vi "WritePFIReport_TempTest.vi"(8 "error in (no error)":errorcluster, 11 "Temp PFI":string[][][](array[string])=[[["11", "12"], ["11", "12"], ["11", "12"], ["11", "12"], ["11", "12"], ["11", "12"], ["11", ""], ["11", ""], ["11", ""], ["11", ""], ["11", ""], ["11", ""], ["", ""], ["", ""]], [["21", "22"], ["21", "22"], ["21", "22"], ["21", "22"], ["21", "22"], ["21", "22"], ["21", "22"], ["21", "22"], ["21", "22"], ["21", "22"], ["21", "22"], ["21", "22"], ["21", "22"], ["21", "22"]]]) -> (0 "error in (no error) 2":errorcluster)   [LabVIEW 2014]
uses:
  Excel(ActiveX)/enumOpenOrCreate.ctl
  Excel(ActiveX)/Excel(ActiveX).lvlib
panel:
  out "deleted portion":string[][](array[string])
  out "array w/ subset deleted":string[][](array[string])
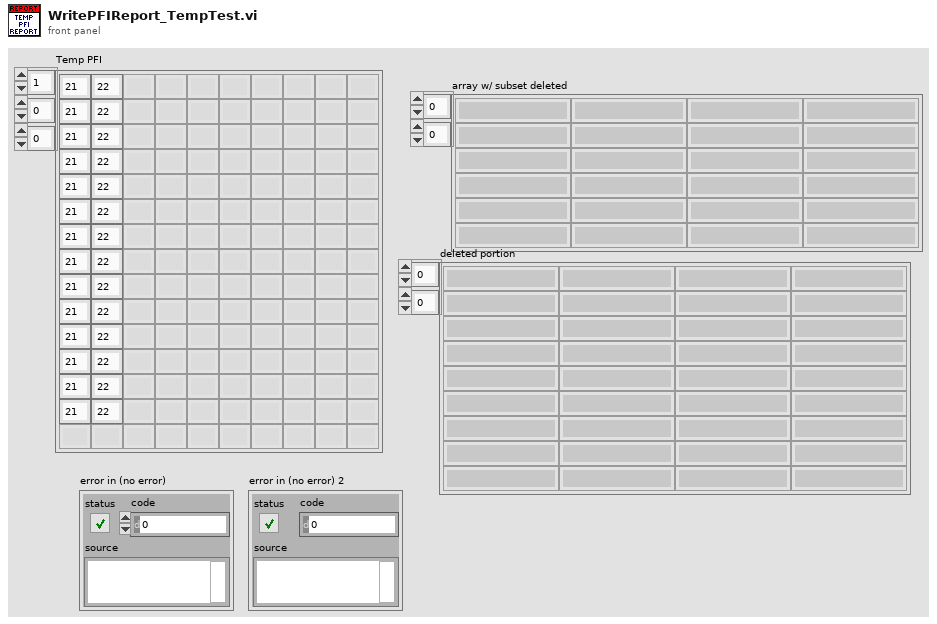
[diagram p1: front panel]
types:
  T1 = typedef "Excel(ActiveX).lvlib/enumOpenOrCreate.ctl" = enum16{"open", "open or create", "create from template"}
  T2 = typedef "Excel(ActiveX).lvlib/ExcelActiveX.ctl" = cluster{"Excel._Application":refnum<k7>, "Application open at start":bool, "Excel._Worksheet":refnum<k7>, "Workbook open at start":bool, "Excel._Workbook":refnum<k7>, "Workbook Path":path, "Worksheet Name":string, "Row":u32, "Col":u32, "Cell":string, "Workbook Name":string}
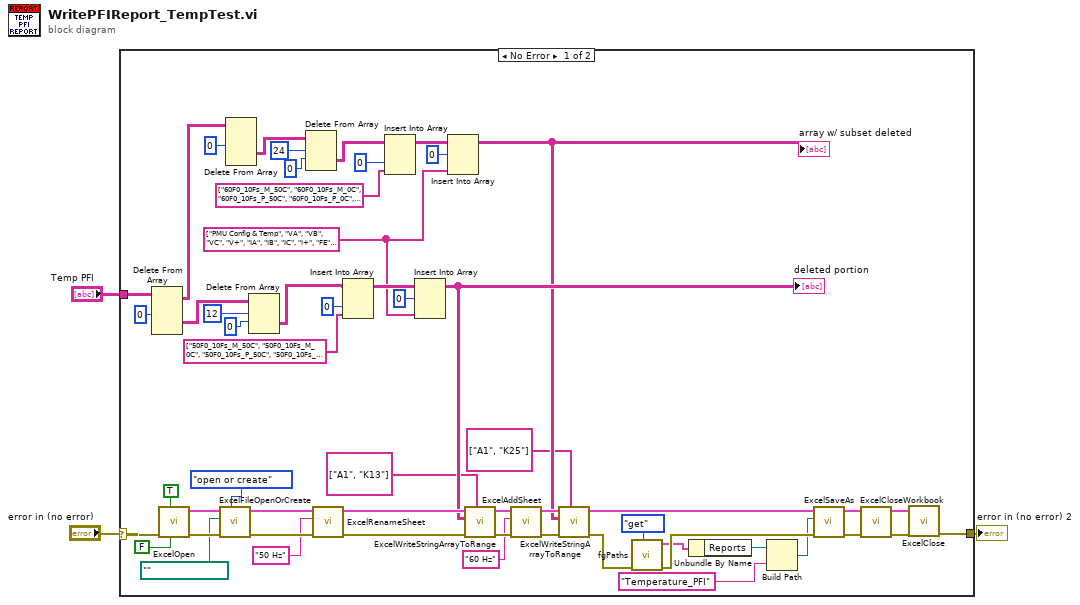
[diagram p0: block diagram]
diagram:
  n1 = case shown="No Error" "error in (no error)" {
    selector: "error in (no error)" -> [w58 w59]
    tunnel: [w12 w59] -> w2
    tunnel: "Temp PFI" -> [w56 _]
    frame No Error {
      w37 = string[] ["PMU Config & Temp", "VA", "VB", "VC", "V+", "IA", "IB", "IC", "I+", "FE", "RFE"]
      n2 = Delete From Array(array=w56, index (dim 0)=0 ("index (page)")) -> (deleted portion=w55:string[][], array with subset deleted=w52:string[][][])  [unwired: 3 in]
      n3 = call "ExcelOpen.vi"("Run Minimized (f)"=FALSE, "Excel visible? (t)"=TRUE, "error in (no error)"=w58) -> ("error out"=w35:errorcluster, "ExcelActiveX"=w34:T2)  [unwired: 7 in]
      n4 = call "ExcelFileOpenOrCreate.vi"("Open or Create"=enumOpenOrCreate."open or create", "error in (no error)"=w35, "Excel file name and path"=path "", "ExcelActiveX in"=w34) -> ("error out"=w31:errorcluster, "ExcelActiveX out"=w32:T2)  [unwired: 6 in]
      n5 = Delete From Array(array=w52, index (dim 0)=0 ("index (page)")) -> (deleted portion=w50:string[][])  [unwired: 3 in, 1 out]
      n6 = Delete From Array(array=w55, length=12, index (row)=0) -> (deleted portion=w48:string[][])  [unwired: 1 in, 1 out]
      n7 = Delete From Array(array=w50, length=24, index (row)=0) -> (deleted portion=w41:string[][])  [unwired: 1 in, 1 out]
      n8 = call "ExcelRenameSheet.vi"("error in (no error)"=w31, "Sheet Name"="50 Hz", "ExcelActiveX"=w32) -> ("error out"=w28:errorcluster, "ExcelActiveX 2"=w27:T2)  [unwired: 7 in]
      n9 = Insert Into Array(array=w48, index (col)=0 ("disabled index (col)"), new element=string[] ["50F0_10Fs_M_50C", "50F0_10Fs_M_0C", "50F0_10Fs_P_50C", "50F0_10Fs_P_0C", "50F0_25Fs_M_50C", "50F0_25Fs_M_0C", "50F0_25Fs_P_50C", "50F0_25Fs_P_0C", "50F0_50Fs_M_50C", "50F0_50Fs_M_0C", "50F0_50Fs_P_50C", "50F0_50Fs_P_0C"]) -> (w39:string[][])  [unwired: 1 in]
      n10 = Insert Into Array(array=w41, index (col)=0 ("disabled index (col)"), new element=string[] ["60F0_10Fs_M_50C", "60F0_10Fs_M_0C", "60F0_10Fs_P_50C", "60F0_10Fs_P_0C", "60F0_12Fs_M_50C", "60F0_12Fs_M_0C", "60F0_12Fs_P_50C", "60F0_12Fs_P_0C", "60F0_15Fs_M_50C", "60F0_15Fs_M_0C", "60F0_15Fs_P_50C", "60F0_15Fs_P_0C", "60F0_20Fs_M_50C", "60F0_20Fs_M_0C", "60F0_20Fs_P_50C", "60F0_20Fs_P_0C", "60F0_30Fs_M_50C", "60F0_30Fs_M_0C", "60F0_30Fs_P_50C", "60F0_30Fs_P_0C", "60F0_60Fs_P_50C", "60F0_60Fs_M_0C", "60F0_60Fs_P_50C", "60F0_60Fs_P_0C"]) -> (w44:string[][])  [unwired: 1 in]
      n11 = Insert Into Array(array=w39, index (row)=0, new element=w37) -> (w26:string[][])  [unwired: 1 in]
      "deleted portion" <- w26
      n12 = Insert Into Array(array=w44, index (row)=0, new element=w37) -> (w18:string[][])  [unwired: 1 in]
      "array w/ subset deleted" <- w18
      n13 = call "ExcelWriteStringArrayToRange.vi"("Range"=string[] ["A1", "K13"], "error in (no error)"=w28, "StringArray"=w26, "ExcelActiveX"=w27) -> ("error out"=w24:errorcluster, "ExcelActiveX"=w23:T2)  [unwired: 6 in]
      n14 = call "ExcelAddSheet.vi"("error in (no error)"=w24, "Sheet Name"="60 Hz", "ExcelActiveX"=w23) -> ("error out"=w20:errorcluster, "ExcelActiveX"=w19:T2)  [unwired: 7 in]
      n15 = call "ExcelWriteStringArrayToRange.vi"("Range"=string[] ["A1", "K25"], "error in (no error)"=w20, "StringArray"=w18, "ExcelActiveX"=w19) -> ("error out"=w10:errorcluster, "ExcelActiveX"=w16:T2)  [unwired: 6 in]
      n16 = call "fgPaths.vi"("cmd"=enum16{"init", "set", "get"}."get", "error in (no error)"=w10) -> ("error out"=w9:errorcluster, "clPaths"=w7:cluster{"Templates":path, "Reports":path})  [unwired: 8 in]
      n17 = Unbundle By Name(w7) -> ("Reports"=w6:path)
      n18 = Build Path(base path=w6, name or relative path="Temperature_PFI") -> (appended path=w4:path)
      n19 = call "ExcelSaveAs.vi"("error in (no error)"=w9, "Path"=w4, "ExcelActiveX"=w16) -> ("error out"=w15:errorcluster, "ExcelActiveX"=w14:T2)  [unwired: 7 in]
      n20 = call "ExcelCloseWorkbook.vi"("error in (no error)"=w15, "ExcelActiveX"=w14) -> ("error out"=w13:errorcluster, "ExcelActiveX"=w11:T2)  [unwired: 8 in]
      n21 = call "ExcelClose.vi"("error in (no error)"=w13, "ExcelActiveX in"=w11) -> ("error out"=w12:errorcluster)  [unwired: 8 in, 1 out]
    }
    frame Error {
    }
  }
  "error in (no error) 2" <- w2
